vi "Get All Destinations.vi"(8 "error in (no error)":errorcluster, 11 "NI_AB_API_Build in":refnum<class "NI_AB_API_Build.lvclass">) -> (0 "error out":errorcluster, 2 "Destinations":T1[](array[typedef]), 3 "NI_AB_API_Build out":refnum<class "NI_AB_API_Build.lvclass">)   [LabVIEW 2020, in "NI_AB_API_Build.lvclass"]
uses:
  <vilib>/AppBuilder/AB_API/Build/NI_AB_API_Build.lvclass
  <vilib>/AppBuilder/AB_API/common/AB_API Destination Data.ctl
  <vilib>/AppBuilder/AB_API/common/AB_API Destination Type.ctl
  <vilib>/AppBuilder/AB_API/Build/NI_AB_API_Build.lvclass/NI_AB_API_Build.ctl
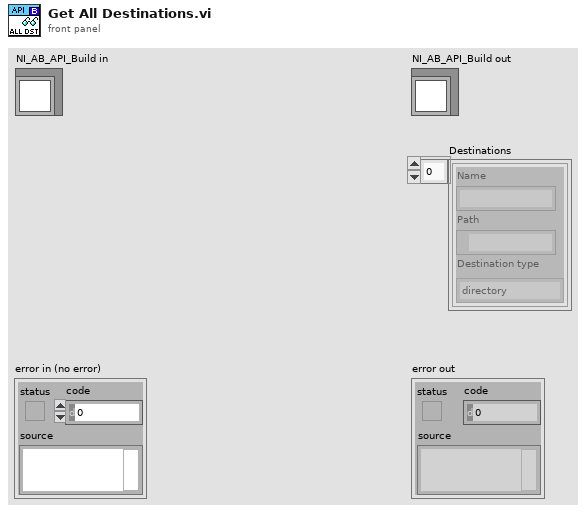
[diagram p1: front panel]
types:
  T1 = typedef "AB_API Destination Data.ctl" = cluster{"Name":string, "Path":path, "Destination type":T2}
  T2 = typedef "AB_API Destination Type.ctl" = enum16{"directory", "directory (preserve hierarchy)", "LLB"}
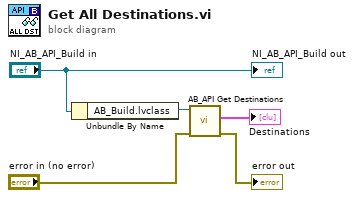
[diagram p0: block diagram]
diagram:
  n1 = Unbundle By Name("NI_AB_API_Build in") -> ("AB_Build.lvclass"=w3:refnum<class "AB_Build.lvclass">)
  n2 = call <vilib>:"AB_API Get Destinations.vi"("error in (no error)"="error in (no error)", "Build in"=w3) -> ("error out"=→"error out":errorcluster, "Destinations"=→"Destinations":T1[])  [unwired: 8 in]
  "NI_AB_API_Build out" <- "NI_AB_API_Build in"
